vi "process data.vi"(6 "Log Data":bool, 8 "Reset":bool, 9 "method":T2={"sampling interval"=0.1, "samples to average"=1, "data interval"=0.0, "stream data"=FALSE, "file path"=refnum, "command"={"command"=enum."Idle", "start time (ms)"=0, "Channel Indices"=[], "Scans per Sample"=1}} {"command"."Scans per Sample" min=1; "data interval" format="%.2f"; "samples to average" min=1 step=1; "sampling interval" format="%.2f"}, 10 "data array":T1[](array[typedef]) {"seconds since 1904" format="%.2f"; "voltage data" format="%.4f"}, 11 "successes":u32) -> (0 "last reading":sgl[](array[numeric]) format="%.2f", 1 "first derivative":sgl[](array[numeric]) format="%.2f", 2 "Time":dbl[](array[numeric]) format="%.2f", 3 "scaled data out":sgl[][](array[numeric]) format="%.5f")   [LabVIEW 2012]
uses:
  DAC apps/support/method.ctl
  DataServer/command cluster.ctl
  DataServer/command.ctl
  DataServer/data send.ctl
panel:
  out "initial time (s)":dbl format="%.1f"
  # "scans\nchannels"
  # "s"
  # "s"
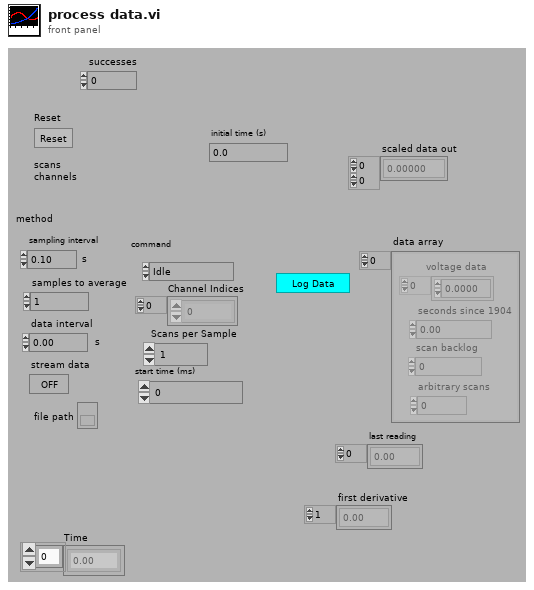
[diagram p1: front panel]
types:
  T1 = typedef "data send.ctl" = cluster{"voltage data":sgl[], "scan backlog":u32, "seconds since 1904":dbl, "arbitrary scans":i32}
  T2 = typedef "method.ctl" = cluster{"sampling interval":sgl, "samples to average":u32, "data interval":sgl, "stream data":bool, "file path":refnum<file>, "command":T3}
  T3 = typedef "command cluster.ctl" = cluster{"command":T4, "start time (ms)":u32, "Channel Indices":i32[], "Scans per Sample":i32}
  T4 = typedef "command.ctl" = enum16{"Idle", "Send Data", "Send 1 Scan", "Logoff"}
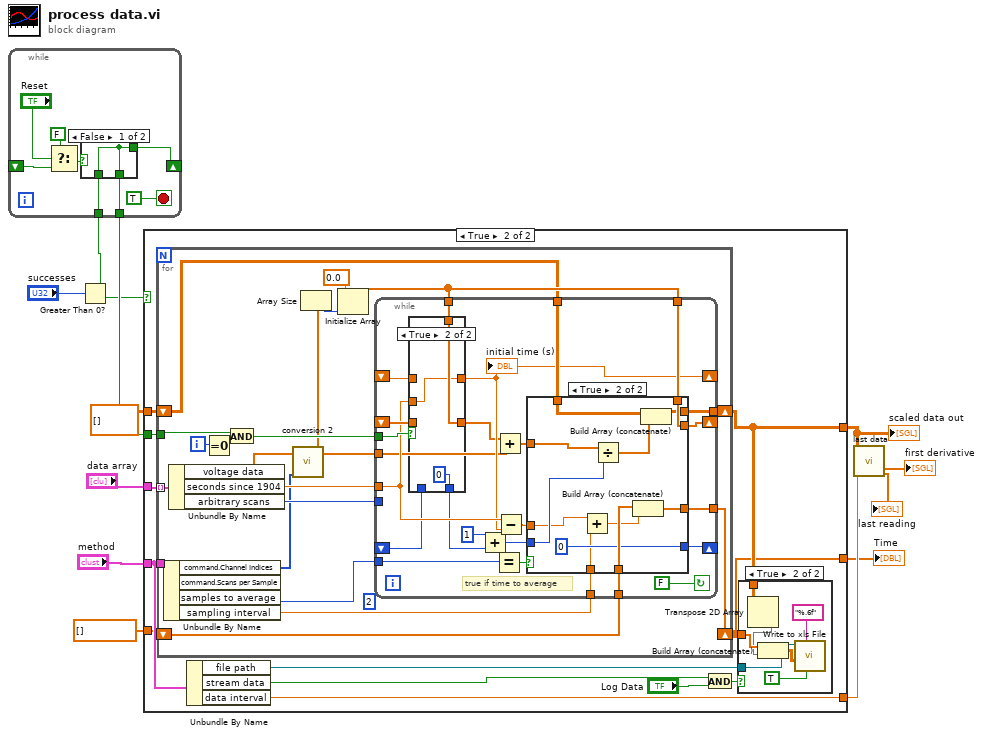
[diagram p0: block diagram]
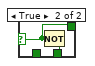
[diagram p2: hidden frame]
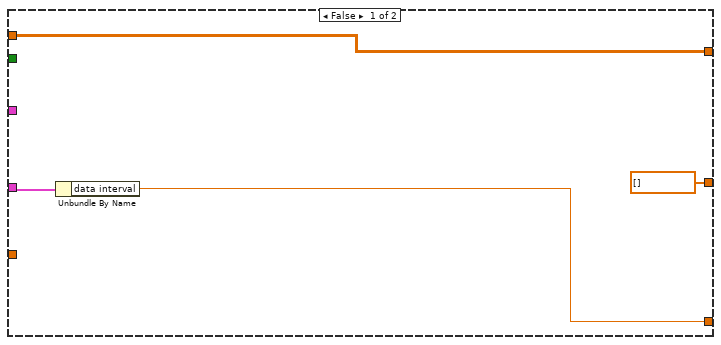
[diagram p3: hidden frame]
diagram:
  n1 = Greater Than 0?(x="successes") -> (x > 0?=w1:bool)
  n2 = while {
    shift-right: [w17] -> _
    shift-left: _ -> [w19]
    tunnel: [w16] -> w2
    tunnel: w1 -> [w15]
    stop <- TRUE stop-if-true
    n3 = Select(t=FALSE, s="Reset", f=w19) -> (s? t:f=w18:bool)
    n4 = case shown="False" w18 {
      selector: w18 -> [_ w22]
      tunnel: [w21 w22] -> w17
      tunnel: w15 -> [w21 _]
      tunnel: [w21 w23] -> w16
      frame False {
      }
      frame True {
        n5 = Not(x=w22) -> (.not. x?=w23:bool)
      }
    }
  }
  n6 = case shown="True" w1 {
    tunnel: [w27 w29] -> w9
    tunnel: sgl[][] [] -> [w27 w39]
    tunnel: "data array" -> [_ w38]
    tunnel: w2 -> [_ w37]
    tunnel: [w25 w31] -> w7
    tunnel: "method" -> [w26 w34]
    tunnel: dbl[] [] -> [_ w30]
    tunnel: [dbl[] [] w28] -> w3
    frame False {
      n7 = Unbundle By Name(w26) -> ("data interval"=w25:sgl)
    }
    frame True {
      n8 = for {
        tunnel: w38 -> [w62] mode=indexing
        shift-right: [w60] -> w29
        shift-left: w39 -> [w61]
        tunnel: w37 -> [w58]
        tunnel: w34 -> [w49]
        shift-right: [w50] -> w28
        shift-left: w30 -> [w51]
        i -> [w59]
        (unwired) i8 2 ("x")
        n9 = Unbundle By Name(w49) -> ("command.Channel Indices"=w48:i32[], "samples to average"=w53:u32, "sampling interval"=w47:sgl)  [unwired: 1 out]
        n10 = Unbundle By Name(w62) -> ("voltage data"=w55:sgl[], "seconds since 1904"=w57:dbl, "arbitrary scans"=w52:i32)
        n11 = Equal To 0?(x=w59) -> (x = 0?=w63:bool)
        n12 = And(x=w58, y=w63) -> (x .and. y?=w56:bool)
        n13 = call "conversion 2.vi"("Channel Indices"=w48, "voltage data"=w55) -> ("calibrated data"=w54:sgl[])  [unwired: 8 in, 1 out]
        n14 = Array Size(array=w54) -> (size(s)=w65:i32)
        n15 = Initialize Array(sgl 0.0, w65) -> (w64:sgl[])
        n16 = while {
          tunnel: [w78] -> w50
          tunnel: w51 -> [w79]
          tunnel: w47 -> [w80]
          tunnel: w52 -> [_]
          tunnel: [w84] -> w60
          tunnel: w61 -> [w85]
          tunnel: w57 -> [w83]
          shift-left: _ -> [w87]
          shift-right: [w82] -> _
          tunnel: w64 -> [w88]
          tunnel: w64 -> [w89]
          tunnel: w56 -> [w86]
          tunnel: w53 -> [w72]
          tunnel: w54 -> [w75]
          shift-left: _ -> [w90]
          shift-right: [w91] -> _
          shift-right: [w73] -> _
          shift-left: _ -> [w70]
          stop <- FALSE continue-if-true
          # "true if time to average"
          n17 = case shown="True" w86 {
            tunnel: [w94 w97] -> w76
            tunnel: w90 -> [w94 _]
            tunnel: w88 -> [_ w97]
            tunnel: w83 -> [_ w96]
            tunnel: [w93 w96] -> w82
            tunnel: w87 -> [w93 _]
            tunnel: [w92 0] -> w69
            tunnel: w70 -> [w92 _]
            frame False {
            }
            frame True {
            }
          }
          "initial time (s)" <- w82
          n18 = Add(x=1, y=w69) -> (x+y=w67:i32)
          n19 = Equal?(x=w67, y=w72) -> (x = y?=w71:bool)
          n20 = Add(x=w76, y=w75) -> (x+y=w74:sgl[])
          n21 = Subtract(x=w83, y=w82) -> (x-y=w81:dbl)
          n22 = case shown="True" w71 {
            tunnel: [w99 w113] -> w91
            tunnel: w89 -> [_ w113]
            tunnel: w85 -> [w101 w112]
            tunnel: [w101 w111] -> w84
            tunnel: w81 -> [_ w103]
            tunnel: w80 -> [_ w102]
            tunnel: w79 -> [w100 w109]
            tunnel: [w100 w108] -> w78
            tunnel: w74 -> [w99 w107]
            tunnel: [w98 0] -> w73
            tunnel: w67 -> [w98 w105]
            frame False {
            }
            frame True {
              n23 = Add(x=w103, y=w102) -> (x+y=w104:dbl)
              n24 = Divide(x=w107, y=w105) -> (x/y=w110:sgl[])
              n25 = Build Array (concatenate)(w109, w104) -> (w108:dbl[])
              n26 = Build Array (concatenate)(w112, w110) -> (w111:sgl[][])
            }
          }
        }
      }
      n27 = Unbundle By Name(w34) -> ("file path"=w32:refnum<file>, "stream data"=w33:bool, "data interval"=w31:sgl)
      n28 = And(x=w33, y="Log Data") -> (x .and. y?=w35:bool)
      n29 = case shown="True" w35 {
        tunnel: w32 -> [_ w45]
        tunnel: w28 -> [_ w44]
        tunnel: w29 -> [_ w43]
        frame False {
        }
        frame True {
          n30 = Transpose 2D Array(2D array=w43) -> (transposed array=w42:sgl[][])
          n31 = Build Array (concatenate)(w44, w42) -> (w41:dbl[][])
          n32 = call "Write to xls File.vi"("transpose? (no:F)"=TRUE ("append to file? (new file:F)"), "format (%.3f)"="%.6f", "2D data"=w41, "refnum"=w45) -> ()  [unwired: 6 in, 2 out]
        }
      }
    }
  }
  "scaled data out" <- w9
  "Time" <- w3
  n33 = call "last data.vi"("data interval"=w7, "calibrated data"=w9) -> ("last reading"=→"last reading":sgl[], "first derivative"=→"first derivative":sgl[])  [unwired: 8 in]
